vi "Write RutaImagenes.vi"(8 "error in (no error)":errorcluster, 10 "RutaImagenes":path, 11 "Simulada in":refnum<class "Simulada.lvclass">) -> (0 "error out":errorcluster, 3 "Simulada out":refnum<class "Simulada.lvclass">)   [LabVIEW 2020, in "Simulada.lvclass"]
uses:
  Simulada.lvclass
  Simulada.lvclass/Simulada.ctl
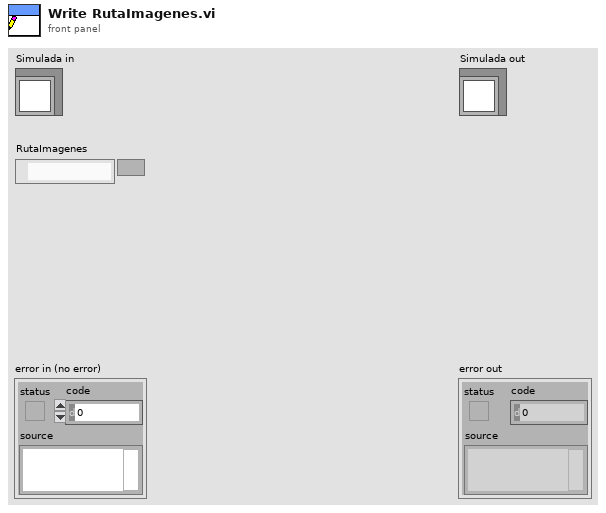
[diagram p1: front panel]
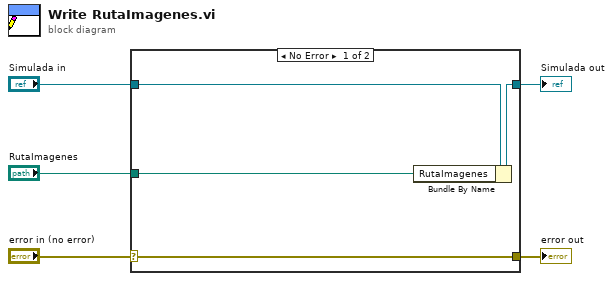
[diagram p0: block diagram]
diagram:
  n1 = case shown="No Error" "error in (no error)" {
    selector: "error in (no error)" -> [w9 w10]
    tunnel: [w9 w10] -> w4
    tunnel: [w7 w11] -> w2
    tunnel: "Simulada in" -> [w8 w11]
    tunnel: "RutaImagenes" -> [w6 _]
    frame No Error {
      n2 = Bundle By Name(cluster=w8, "RutaImagenes"=w6) -> (w7:refnum<class "Simulada.lvclass">)
    }
    frame Error {
    }
  }
  "error out" <- w4
  "Simulada out" <- w2
